vi "Compressor Control.vi"() -> ()   [LabVIEW 2016]
doc: "This VI hosts two shared variables that can be accessed by a variety of client VIs. Shared Variables are typically used for monitoring lossy data, like memory usage, temperature data, etc."
uses:
  CM_Virtual_Panel_LV9_0.llb/Com_Set_AX.ctl
  <vilib>/Instr/_visa.llb/VISA Configure Serial Port (Serial Instr).vi
panel:
  out "power":dbl(graph)
  out "Heater Power":string
  out "Cold head pressure":string
  out "Unit":string="°C"
  out "Cold Head T":dbl=24.81
  out "Motor Current (A)":dbl(knob) scale=0.0..50.0
  out "Compressor Status":bool
  out "Overide status":bool
  out "Comp ON":bool
  out "?":cluster{dbl, dbl, dbl}(slide) scale=32.0..120.0
  out "?":cluster{dbl, dbl, dbl}(slide) scale=32.0..220.0
  out "?":cluster{dbl, dbl, dbl}(slide) scale=32.0..125.0
  out "?":cluster{dbl, dbl, dbl}(slide) scale=32.0..85.0
  out "DP":dbl(knob) scale=0.0..265.0
  in  "CM Tab Control":enum32{"Configuration", "Status"}(tab)
  in  "COM PORT SETUP":T1={"Com Port #"=2, "Timeout(ms)"=500, "Baud"=115200, "Slave Address"=16, "LinkMode"=enum."SMDP-II:Checksum and stamp", "Num Retries"=0} {"Slave Address" min=16; "Com Port #" min=1}
  in  "Data Read Length":u32
  in  "Pressure Monitor Port":refnum<visa-resource-name>
  in  "Command read length":u32
  in  "Separation length":i32
  out "error out":errorcluster
  out "data feedback":string
  out "command feedback":string
  out "Gauge":cluster{dbl, dbl, dbl, dbl, dbl, dbl}(knob)={0.0, 0.0, -0.1, 0.0, 0.0, 0.0} scale=0.0..400.0
  in  "Additel 681 Tab Control":enum32{"Gauge Control", "Status"}(tab)
  in  "Zero Reading":bool
  in  "Cancel Zero reading":bool
  out "Gauge battery Voltage":dbl
  in  "Read":bool
  in  "Enable light control":bool
  in  "Gauge light":bool
  in  "Abort monitoring":bool
  out "Battery status":bool
  out "yellow":bool
  out "orange":bool
  out "red":bool
  in  "voltage read length":u32=25
  out "Voltage feedback":string
  in  "monitor 2 read length":u32=25
  out "monitor 2 feedback":string
  in  "monitor 1 read length":u32=25
  out "Monitor 1 feedback":string
  out "Pump 1 switch":bool
  out "Pump 2 switch":bool
  out "Unit":string="°C"
  out "He pressure":dbl=1.198
  out "Monitor 1":cluster{"He pressure":dbl, "pressure":dbl}(graph)
  in  "Reading 1":string(combo)="255:R:MRMD"
  out "Vapor Temp":dbl=24.81
  out "Monitor 2":dbl(graph)=24.81
  in  "Reading 2":string(combo)="255:R:OTEMP"
  out "Unit":string
  out "Monitor 3":dbl(graph)=0.006479277826451128
  out "Pump 2":dbl=0.006479277826451128 format="%#_2e"
  out "Monitor 4":T2(graph)
  out "Unit":string="Torr"
  out "Pump 1":dbl=0.006515415732577395 format="%#_2e"
  in  "Compressor Relay Control":enum32{"Normal", "Overide"}(tab)
  in  "Pressure Upper Limit":dbl=6.0
  out "Helium Overpressure":bool
  in  "Pressure Lower Limit":dbl=1.0
  in  "Set Relay voltage":dbl(slide)=9.0 scale=0.0..10.0
  out "Numeric 2":dbl=9.0
  out "Helium underpressure":bool
  in  "Compressor On":bool caption="Compressor Ona"
  # "Additel Pressure Gauge"
  # "Cryomech Liquefier"
  # "Pressure (Psi)"
  # "Cryomech Control"
  # "max"
  # "now"
  # "min"
  # "Coolant Supply"
  # "Coolant Return"
  # "Exchage Helium"
  # "Motor Oil"
  # "Temperature °C"
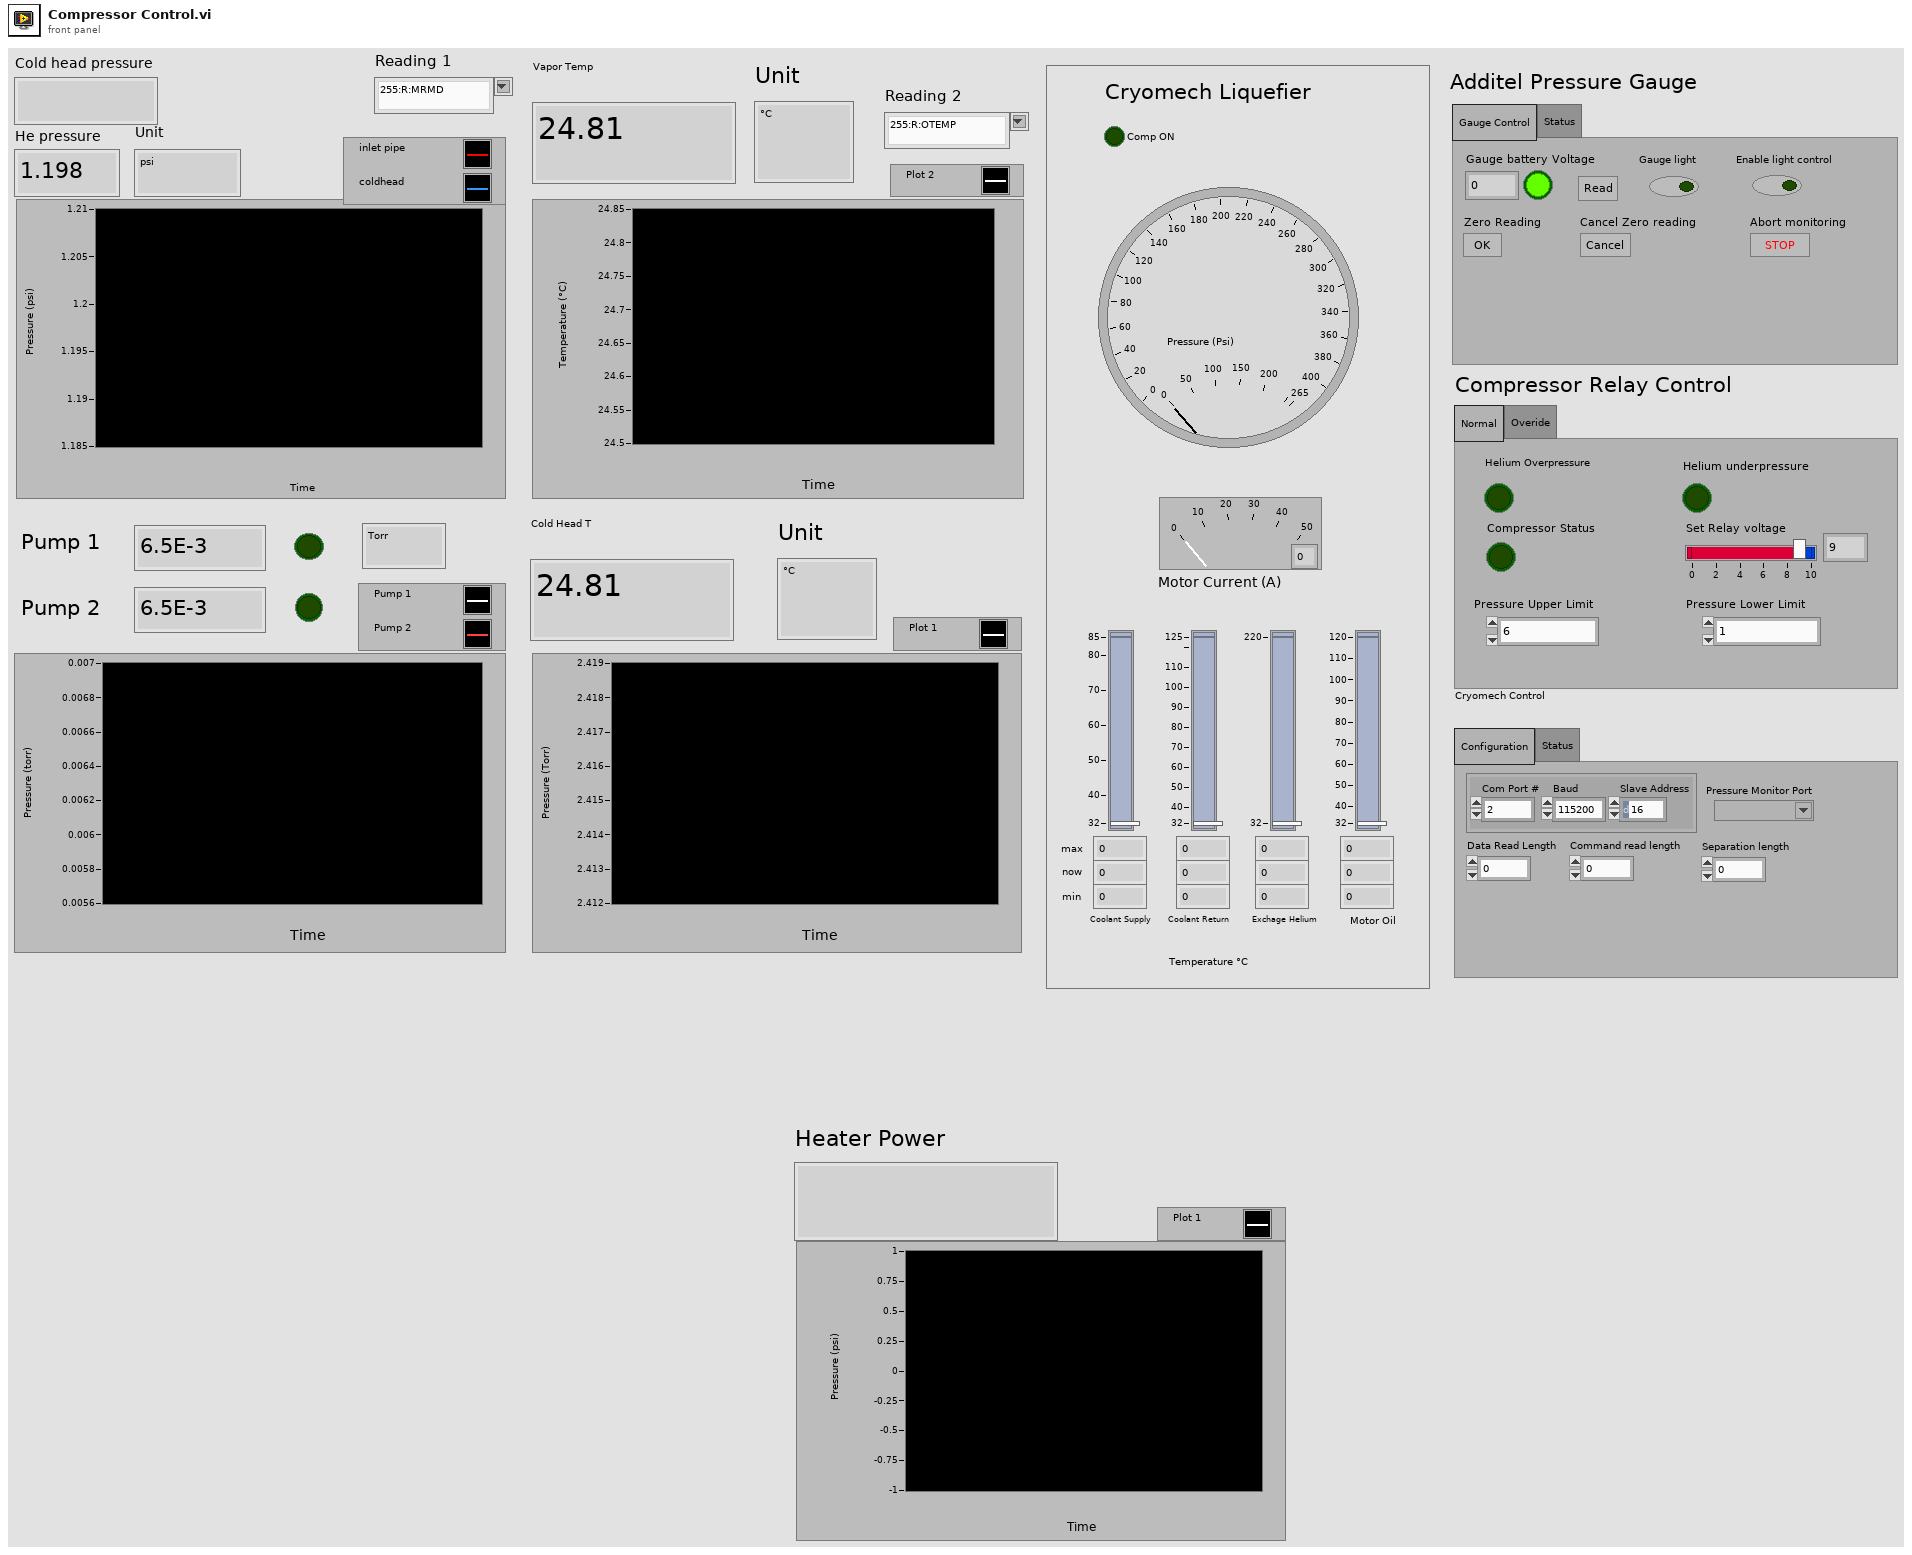
[diagram p1: front panel]
types:
  T1 = typedef "Com_Set_AX.ctl" = cluster{"Com Port #":u8, "Timeout(ms)":u32, "Baud":u32, "Slave Address":u8, "LinkMode":enum16{"SMDP-I:Checksum, no stamp", "SMDP-II:Checksum and stamp", "Sycon Protocol"}, "Num Retries":u8}
  T2 = cluster{"Output Variable 1":dbl, "Output Variable 2":dbl}
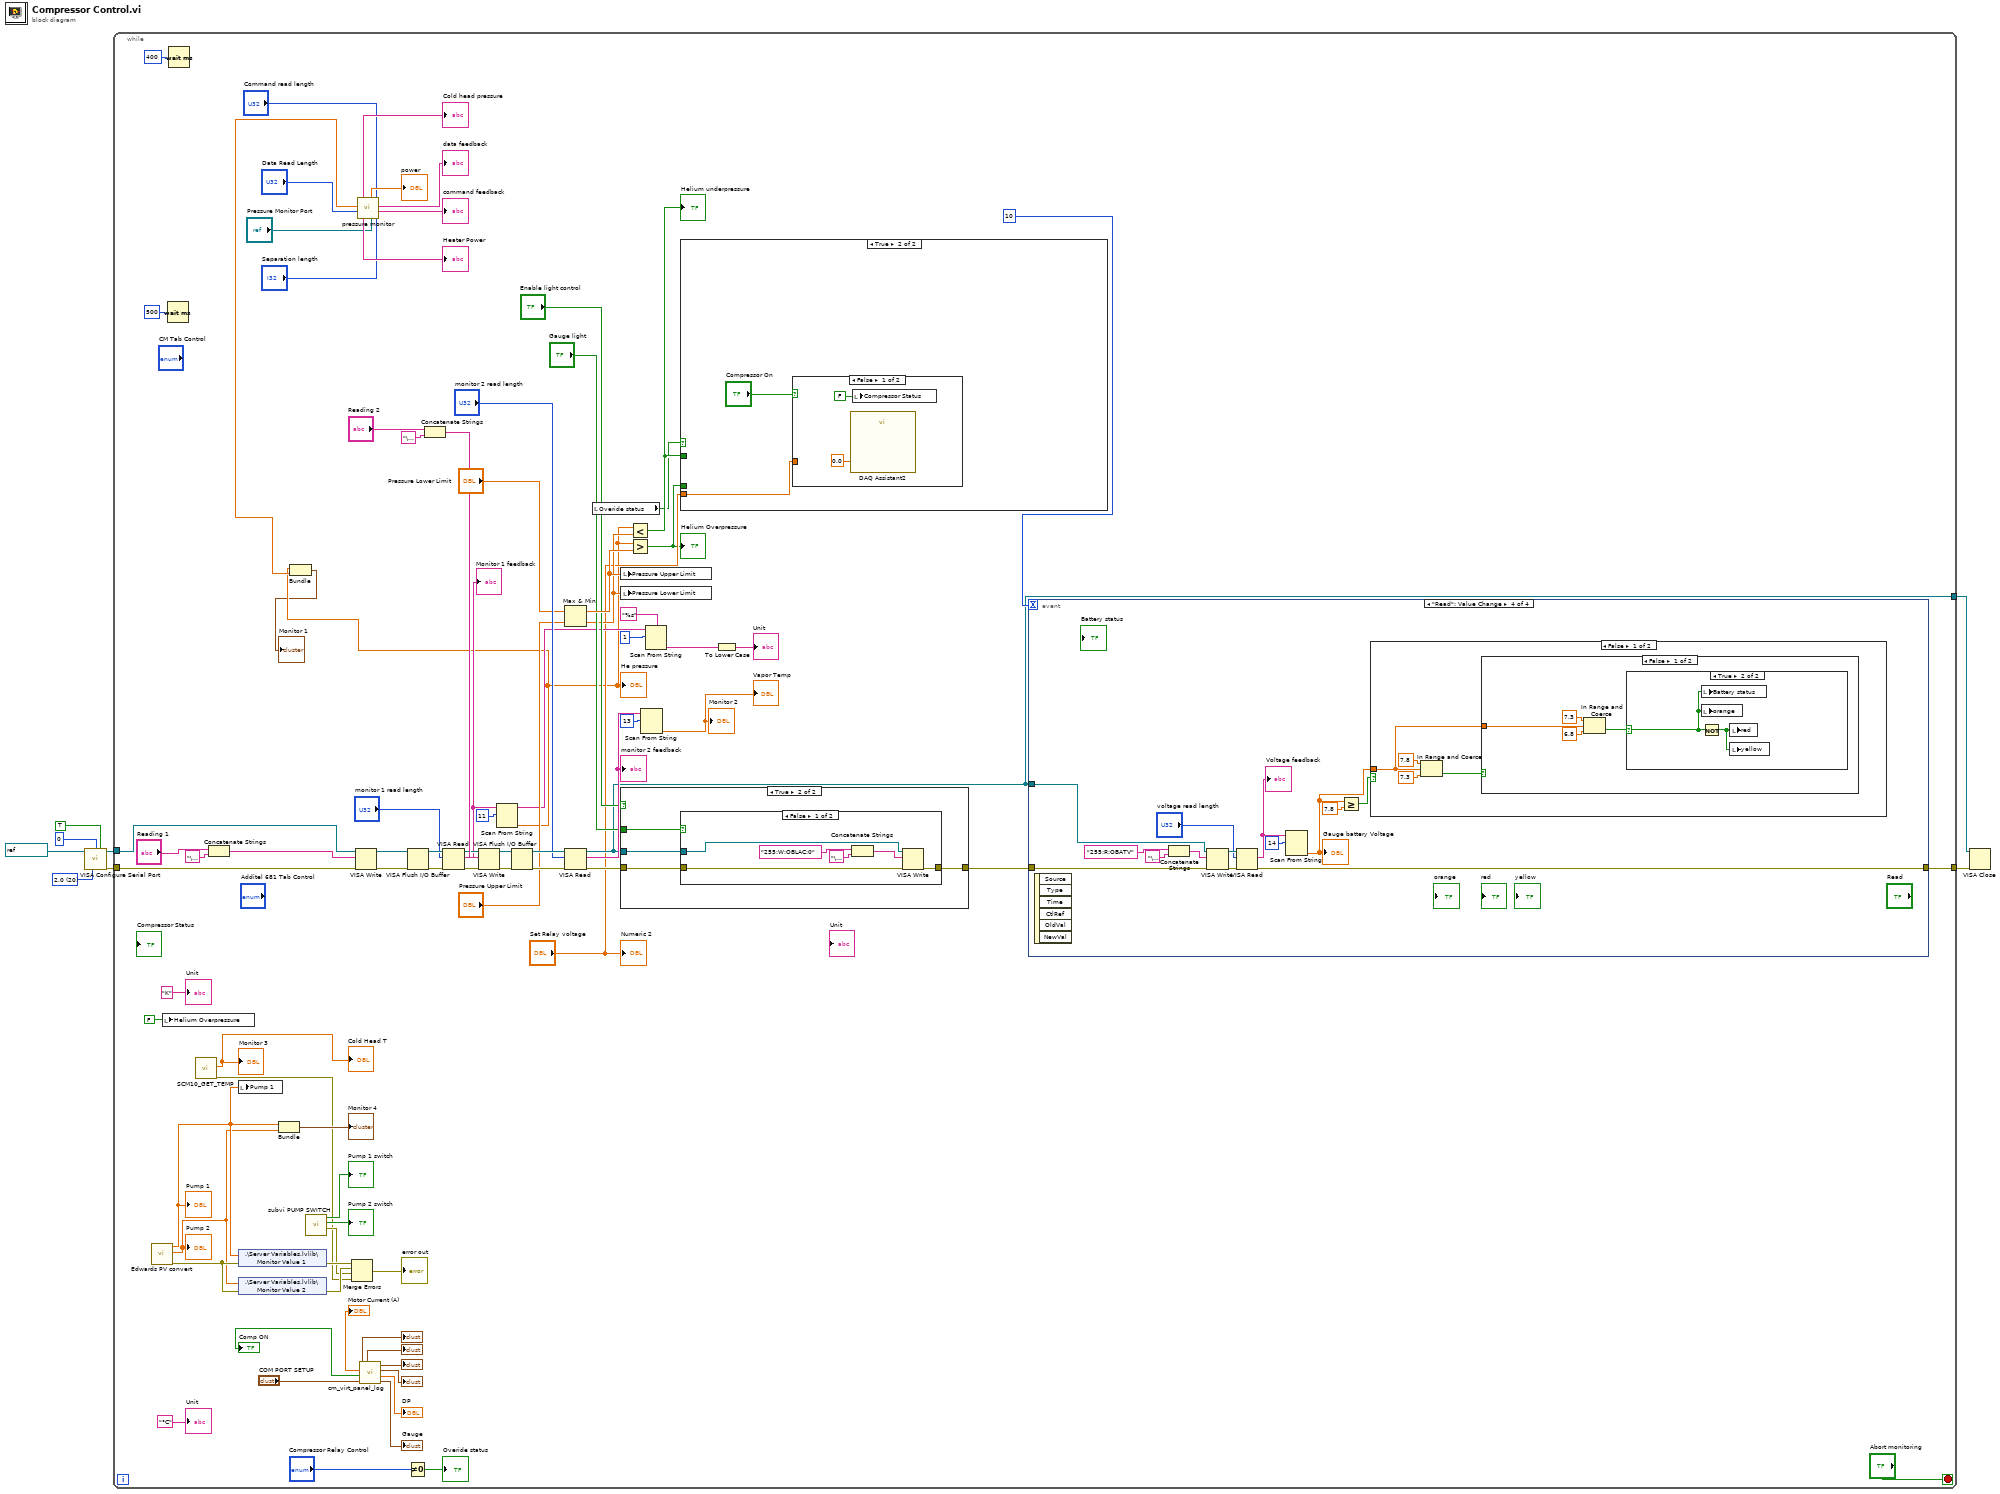
[diagram p0: block diagram]
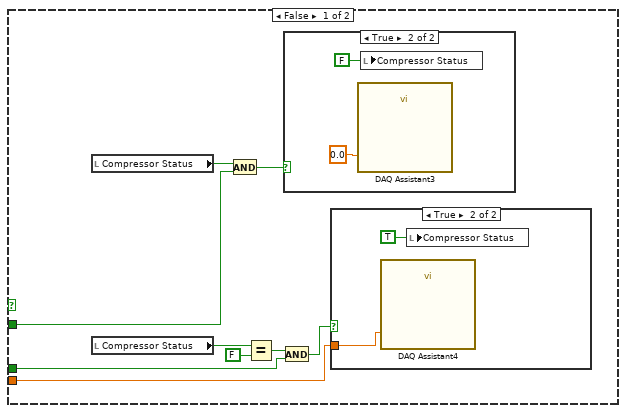
[diagram p2: hidden frame]
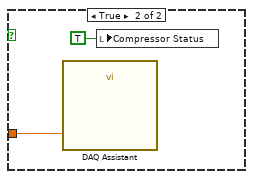
[diagram p5: hidden frame]
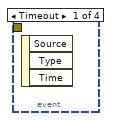
[diagram p6: hidden frame]
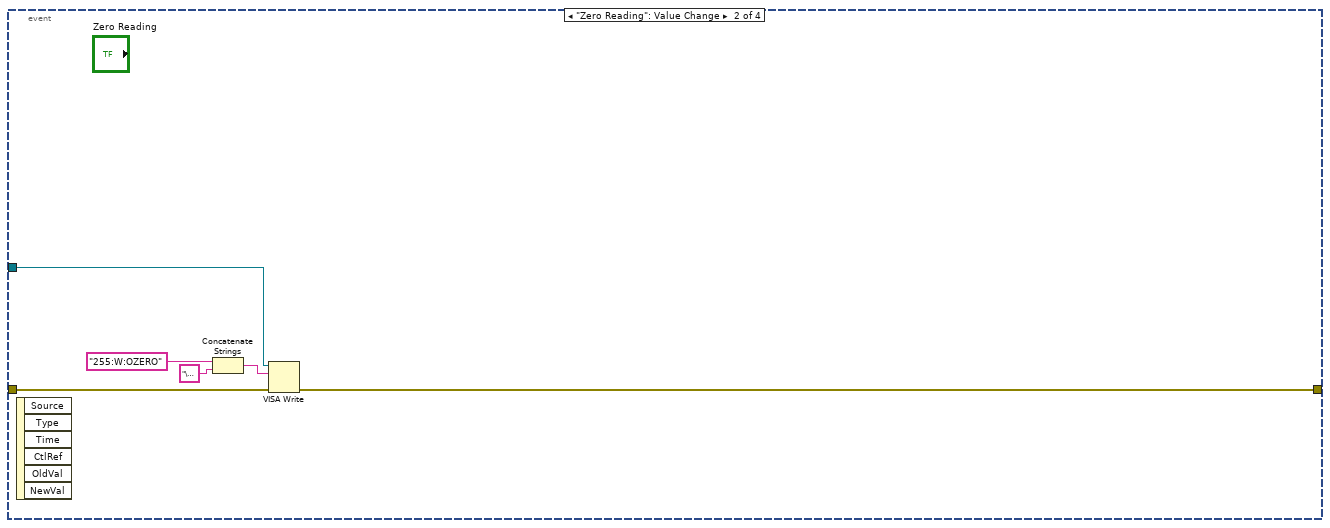
[diagram p7: hidden frame]
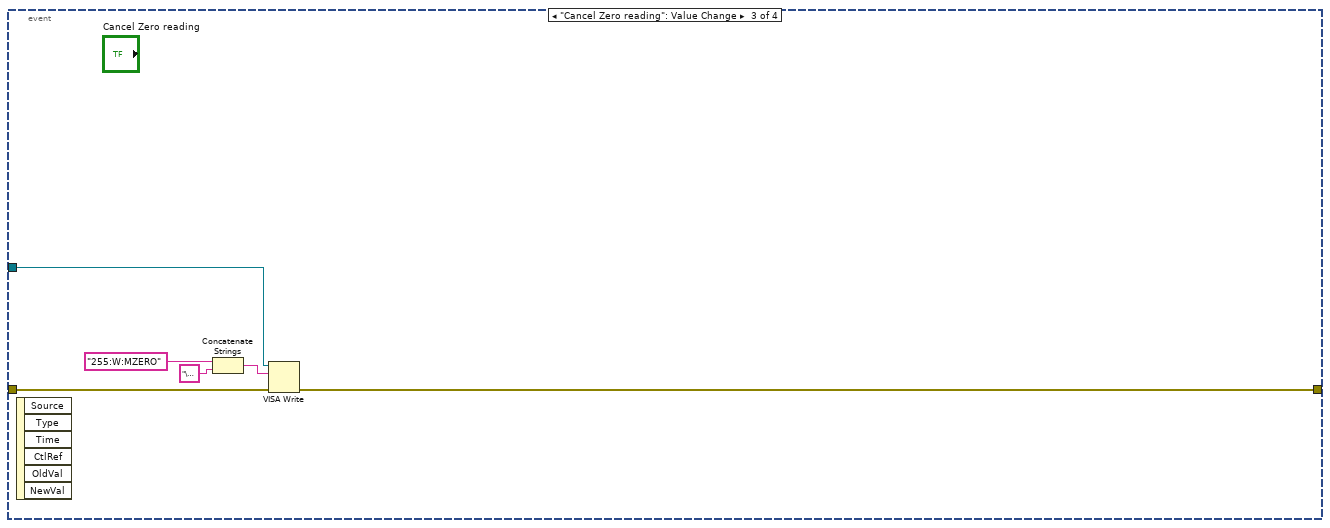
[diagram p8: hidden frame]
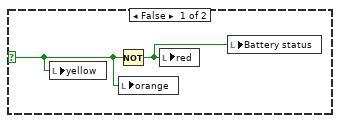
[diagram p9: hidden frame]
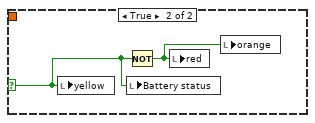
[diagram p10: hidden frame]
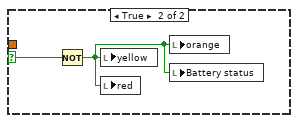
[diagram p11: hidden frame]
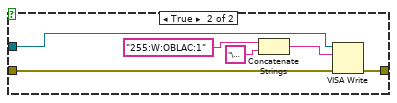
[diagram p13: hidden frame]
diagram:
  w5 = u16 20 items=["1.0"=10, "1.5"=15, "2.0"=20] ("stop bits (10: 1 bit)")
  n1 = call-poly "VISA Configure Serial Port"("VISA resource name"=refnum<visa-resource-name> "COM3", "termination char\n(0xA = '\\n' = LF)"=u8 0 ("termination char\n(0xA = '\\n' = LF)"), "Enable Termination\nChar (T)"=TRUE ("Enable Termination\nChar (T)"), "stop bits (10: 1 bit)"=w5) -> ("VISA resource name out"=w3:refnum<visa-resource-name>, "error out"=w4:errorcluster)  [unwired: 10 in]
  n2 = while {
    tunnel: [w62] -> w2
    tunnel: w4 -> [w34]
    tunnel: w3 -> [w68]
    tunnel: [w61] -> w1
    stop <- "Abort monitoring" stop-if-true
    n3 = call "Edwards PV convert.vi"() -> ("error out"=w37:errorcluster, "Output Variable 2"=w25:dbl, "Output Variable 1"=w26:dbl)  [unwired: 9 in]
    "Pump 2" <- w25
    "Pump 1" <- w26
    n4 = local write "Helium Overpressure"(FALSE ("Helium Overpressure")) -> ()
    n5 = Wait (ms)(milliseconds to wait=u32 500) -> ()  [unwired: 1 out]
    n6 = Wait (ms)(milliseconds to wait=u32 400) -> ()  [unwired: 1 out]
    n7 = call "SCM10_GET_TEMP.vi"() -> ("ERR OUT"=w23:errorcluster, "Temperature (K)"=→"Monitor 3" →"Cold Head T":dbl)  [unwired: 9 in, 1 out]
    n8 = Concatenate Strings("Reading 1", "\u0000") -> (w94:string)
    n9 = local write "Pump 1"(w26) -> ()
    n10 = shared-variable ".\\Server Variables.lvlib\\Monitor Value 1"(w26, error in=w37) -> (error out=w36:errorcluster)
    n11 = shared-variable ".\\Server Variables.lvlib\\Monitor Value 2"(w25, error in=w37) -> (error out=w35:errorcluster)
    n12 = Bundle("Output Variable 1"=w26, "Output Variable 2"=w25) -> (→"Monitor 4":T2)  [unwired: 1 in]
    n13 = call "subvi PUMP SWITCH.vi"() -> ("error out"=w33:errorcluster, "data out"=→"Pump 2 switch":bool, "data out 2"=→"Pump 1 switch":bool)  [unwired: 9 in]
    n14 = Merge Errors(w36, w35, w33, w23) -> (→"error out":errorcluster)
    n15 = VISA Write(VISA resource name=w68, write buffer=w94, error in (no error)=w34) -> (VISA resource name out=w90:refnum<visa-resource-name>, error out=w92:errorcluster)  [unwired: 1 out]
    n16 = call "pressure monitor.vi"("Data Read Length"="Data Read Length", "Pressure Monitor Port"="Pressure Monitor Port", "Command read length"="Command read length", "Separation length"="Separation length") -> ("Cold head pressure"=→"Cold head pressure":string, "pressure"=w11:dbl, "Heater Power"=→"Heater Power":string, "power"=→"power":dbl, "data feedback"=→"data feedback":string, "command feedback"=→"command feedback":string)
    n17 = call "cm_virt_panel_log.vi"("COM PORT SETUP"="COM PORT SETUP") -> ("Gauge"=→"Gauge":cluster{dbl, dbl, dbl, dbl, dbl, dbl}, "DP"=→"DP":dbl, "H2O IN"=→"?":cluster{dbl, dbl, dbl}, "H2O OUT"=→"?":cluster{dbl, dbl, dbl}, "He GAS"=→"?":cluster{dbl, dbl, dbl}, "Comp ON"=→"Comp ON":bool, "Motor Amps"=→"Motor Current (A)":dbl, "OIL TEMP"=→"?":cluster{dbl, dbl, dbl})
    n18 = VISA Flush I/O Buffer(VISA resource name=w90, error in (no error)=w92) -> (VISA resource name out=w91:refnum<visa-resource-name>, error out=w87:errorcluster)  [unwired: 1 in]
    n19 = Not Equal To 0?(x="Compressor Relay Control") -> (x != 0?=→"Overide status":bool)
    n20 = Concatenate Strings("Reading 2", "\u0000") -> (w83:string)
    n21 = VISA Read(VISA resource name=w91, byte count="monitor 1 read length", error in (no error)=w87) -> (VISA resource name out=w73:refnum<visa-resource-name>, read buffer=w59:string, error out=w72:errorcluster)  [unwired: 1 out]
    "Monitor 1 feedback" <- w59
    n22 = VISA Write(VISA resource name=w73, write buffer=w83, error in (no error)=w72) -> (VISA resource name out=w79:refnum<visa-resource-name>, error out=w81:errorcluster)  [unwired: 1 out]
    n23 = Scan From String(input string=w59, initial scan location=u32 11) -> (remaining string=w57:string, output 1=w10:dbl)  [unwired: 3 in, 2 out]
    "He pressure" <- w10
    n24 = Bundle("He pressure"=w10, "pressure"=w11) -> (→"Monitor 1":cluster{"He pressure":dbl, "pressure":dbl})  [unwired: 1 in]
    n25 = VISA Flush I/O Buffer(VISA resource name=w79, error in (no error)=w81) -> (VISA resource name out=w80:refnum<visa-resource-name>, error out=w75:errorcluster)  [unwired: 1 in]
    n26 = Max & Min(x="Pressure Lower Limit", y="Pressure Upper Limit") -> (max(x,y)=w69:dbl, min(x,y)=w53:dbl)
    n27 = VISA Read(VISA resource name=w80, byte count="monitor 2 read length", error in (no error)=w75) -> (VISA resource name out=w62:refnum<visa-resource-name>, read buffer=w77:string, error out=w65:errorcluster)  [unwired: 1 out]
    "monitor 2 feedback" <- w77
    n28 = local read "Overide status"() -> (w29:bool)
    n29 = local write "Pressure Upper Limit"(w69) -> ()
    n30 = local write "Pressure Lower Limit"(w53) -> ()
    n31 = case shown="True" "Enable light control" {
      tunnel: "Gauge light" -> [_ w160]
      tunnel: w65 -> [w156 w159]
      tunnel: [w156 w158] -> w60
      tunnel: w62 -> [_ w157]
      frame False {
      }
      frame True {
        n32 = case shown="False" w160 {
          tunnel: w157 -> [w163 w172]
          tunnel: [w162 w168] -> w158
          tunnel: w159 -> [w161 w167]
          frame False {
            n33 = Concatenate Strings("255:W:OBLAC:0" ("string"), "\u0000" ("string")) -> (w164:string)
            n34 = VISA Write(VISA resource name=w163, write buffer=w164, error in (no error)=w161) -> (error out=w162:errorcluster)  [unwired: 2 out]
          }
          frame True {
            n35 = Concatenate Strings("255:W:OBLAC:1" ("string"), "\u0000" ("string")) -> (w169:string)
            n36 = VISA Write(VISA resource name=w172, write buffer=w169, error in (no error)=w167) -> (error out=w168:errorcluster)  [unwired: 2 out]
          }
        }
      }
    }
    n37 = Less?(x=w10, y=w53) -> (x < y?=w38:bool)
    "Helium underpressure" <- w38
    n38 = Greater?(x=w10, y=w69) -> (0:w39:bool)
    "Helium Overpressure" <- w39
    n39 = Scan From String(input string=w77, initial scan location=u32 13) -> (output 1=→"Vapor Temp" →"Monitor 2":dbl)  [unwired: 3 in, 3 out]
    n40 = Scan From String(format string="%s", input string=w57, initial scan location=u32 1) -> (output 1=w55:string)  [unwired: 2 in, 3 out]
    n41 = case shown="True" w29 {
      tunnel: "Set Relay voltage" -> [w100 w108]
      tunnel: w39 -> [w96 _]
      tunnel: w38 -> [w95 _]
      frame False {
        n42 = local read "Compressor Status"() -> (w103:bool)
        n43 = local read "Compressor Status"() -> (w99:bool)
        n44 = And(x=w103, y=w95) -> (x .and. y?=w102:bool)
        n45 = Equal?(x=w99, y=FALSE) -> (x = y?=w97:bool)
        n46 = And(x=w97, y=w96) -> (x .and. y?=w101:bool)
        n47 = case shown="True" w102 {
          frame False {
          }
          frame True {
            n48 = call "DAQ Assistant3"("data"=0.0) -> ()  [unwired: 17 in, 2 out]
            n49 = local write "Compressor Status"(FALSE ("Compressor Status")) -> ()
          }
        }
        n50 = case shown="True" w101 {
          tunnel: w100 -> [_ w107]
          frame False {
          }
          frame True {
            n51 = call "DAQ Assistant4"("data"=w107) -> ()  [unwired: 17 in, 2 out]
            n52 = local write "Compressor Status"(TRUE ("Compressor Status")) -> ()
          }
        }
      }
      frame True {
        n53 = case shown="False" "Compressor On" {
          tunnel: w108 -> [_ w113]
          frame False {
            n54 = call "DAQ Assistant2"("data"=0.0) -> ()  [unwired: 17 in, 2 out]
            n55 = local write "Compressor Status"(FALSE ("Compressor Status")) -> ()
          }
          frame True {
            n56 = call "DAQ Assistant"("data"=w113) -> ()  [unwired: 17 in, 2 out]
            n57 = local write "Compressor Status"(TRUE ("Compressor Status")) -> ()
          }
        }
      }
    }
    n58 = To Lower Case(string=w55) -> (all lower case string=→"Unit":string)
    n59 = event shown="[3] \"Read\": Value Change" {
      selector: _ -> [_ _ _ _]
      dyn-events: _ -> [_ _ _ _]
      timeout: 10 -> [_ _ _ _]
      tunnel: w62 -> [_ w114 w121 w131]
      tunnel: [_ w115 w120 w130] -> w61
      tunnel: w60 -> [_ w116 w122 w127]
      event Timeout {
        n60 = event-data() -> ()  [unwired: 1 in, 3 out]
      }
      event "Zero Reading": Value Change {
        n61 = event-data() -> ()  [unwired: 1 in, 6 out]
        n62 = Concatenate Strings("255:W:OZERO" ("string"), "\u0000" ("string")) -> (w117:string)
        n63 = VISA Write(VISA resource name=w114, write buffer=w117, error in (no error)=w116) -> (error out=w115:errorcluster)  [unwired: 2 out]
      }
      event "Cancel Zero reading": Value Change {
        n64 = event-data() -> ()  [unwired: 1 in, 6 out]
        n65 = Concatenate Strings("255:W:MZERO" ("string"), "\u0000" ("string")) -> (w125:string)
        n66 = VISA Write(VISA resource name=w121, write buffer=w125, error in (no error)=w122) -> (error out=w120:errorcluster)  [unwired: 2 out]
      }
      event "Read": Value Change {
        n67 = event-data() -> ()  [unwired: 1 in, 6 out]
        n68 = Concatenate Strings("255:R:OBATV" ("string"), "\u0000" ("string")) -> (w137:string)
        n69 = VISA Write(VISA resource name=w131, write buffer=w137, error in (no error)=w127) -> (VISA resource name out=w135:refnum<visa-resource-name>, error out=w136:errorcluster)  [unwired: 1 out]
        n70 = VISA Read(VISA resource name=w135, byte count="voltage read length", error in (no error)=w136) -> (read buffer=w133:string, error out=w130:errorcluster)  [unwired: 2 out]
        "Voltage feedback" <- w133
        n71 = Scan From String(input string=w133, initial scan location=u32 14) -> (output 1=w126:dbl)  [unwired: 3 in, 3 out]
        "Gauge battery Voltage" <- w126
        n72 = Greater Or Equal?(x=w126, y=7.8) -> (x >= y?=w128:bool)
        n73 = case shown="False" w128 {
          selector: w128 -> [_ w155]
          tunnel: w126 -> [w140 _]
          frame False {
            n74 = In Range and Coerce(upper limit=7.8, x=w140, lower limit=7.3) -> (In Range?=w141:bool)  [unwired: 1 out]
            n75 = case shown="False" w141 {
              selector: w141 -> [_ w153]
              tunnel: w140 -> [w147 _]
              frame False {
                n76 = In Range and Coerce(upper limit=7.3, x=w147, lower limit=6.8) -> (In Range?=w144:bool)  [unwired: 1 out]
                n77 = case shown="True" w144 {
                  selector: w144 -> [w149 w151]
                  frame False {
                    n78 = local write "yellow"(w149) -> ()
                    n79 = Not(x=w149) -> (.not. x?=w148:bool)
                    n80 = local write "orange"(w149) -> ()
                    n81 = local write "red"(w148) -> ()
                    n82 = local write "Battery status"(w148) -> ()
                  }
                  frame True {
                    n83 = Not(x=w151) -> (.not. x?=w150:bool)
                    n84 = local write "Battery status"(w151) -> ()
                    n85 = local write "orange"(w151) -> ()
                    n86 = local write "red"(w150) -> ()
                    n87 = local write "yellow"(w150) -> ()
                  }
                }
              }
              frame True {
                n88 = local write "yellow"(w153) -> ()
                n89 = Not(x=w153) -> (.not. x?=w152:bool)
                n90 = local write "Battery status"(w153) -> ()
                n91 = local write "red"(w152) -> ()
                n92 = local write "orange"(w152) -> ()
              }
            }
          }
          frame True {
            n93 = Not(x=w155) -> (.not. x?=w154:bool)
            n94 = local write "yellow"(w154) -> ()
            n95 = local write "red"(w154) -> ()
            n96 = local write "orange"(w154) -> ()
            n97 = local write "Battery status"(w154) -> ()
          }
        }
      }
    }
    "Unit" <- "°C" ("Unit")
    "Numeric 2" <- "Set Relay voltage"
    "Unit" <- "K" ("Unit")
  }
  n98 = VISA Close(VISA resource name=w2, error in (no error)=w1) -> ()  [unwired: 1 out]
